vi "서보모터.vi"() -> ()   [LabVIEW 2018]
uses:
  <vilib>/DAQmx/write.llb/DAQmx Write (Counter Frequency 1Chan 1Samp).vi
  <vilib>/DAQmx/create/channels.llb/DAQmx Create Channel (CO-Pulse Generation-Frequency).vi
  <vilib>/DAQmx/configure/timing.llb/DAQmx Timing (Implicit).vi
  <vilib>/DAQmx/miscellaneous.llb/DAQmx Fill In Error Info.vi
panel:
  out "Duty Cycle":dbl
  in  "정지 버튼":bool
  in  "다이얼":dbl(knob)=0.5 caption="주기 점유율" scale=0.01..0.9
  in  "frequency":dbl=1.0 caption="주파수" format="%.6f"
  in  "initial delay":dbl caption="초기 지연" format="%.6f"
  in  "idle state":i32(ring)=10214 caption="유휴 상태" items=["하이"=10192, "로우"=10214]
  in  "counter":tag caption="카운터"
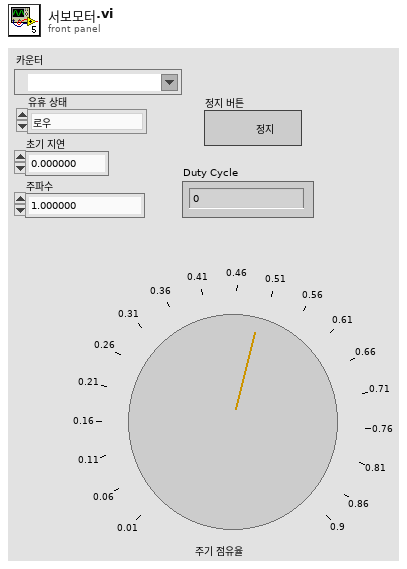
[diagram p1: front panel]
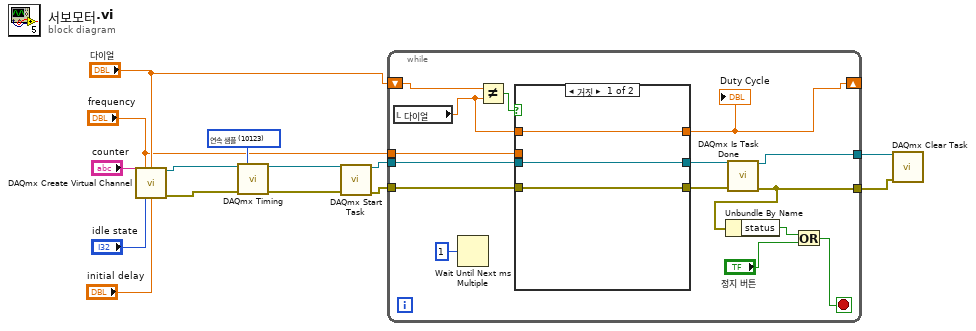
[diagram p0: block diagram]
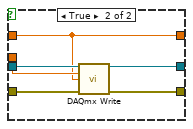
[diagram p2: hidden frame]
diagram:
  w7 = 10123 items=["유한 샘플"=10178, "연속 샘플"=10123, "하드웨어 타이밍에 의한 단일 포인트"=12522] ("sample mode")
  n1 = call-poly <vilib>:"DAQmx Create Virtual Channel.vi"("frequency"="frequency", "duty cycle"="다이얼", "counter"="counter", "idle state"="idle state", "initial delay"="initial delay") -> ("task out"=w14:refnum<k21>, "error out"=w13:errorcluster)  [unwired: 9 in]
  n2 = call-poly <vilib>:"DAQmx Timing.vi"("task/channels in"=w14, "sample mode"=w7, "error in"=w13) -> ("task out"=w11:refnum<k21>, "error out"=w12:errorcluster)  [unwired: 11 in]
  n3 = call <vilib>:"DAQmx Start Task.vi"("task/channels in"=w11, "error in"=w12) -> ("task out"=w4:refnum<k21>, "error out"=w3:errorcluster)  [unwired: 12 in]
  n4 = while {
    tunnel: [w29] -> w6
    tunnel: [w19] -> w5
    tunnel: w4 -> [w28]
    tunnel: w3 -> [w27]
    shift-right: [w21] -> _
    shift-left: "다이얼" -> [w24]
    tunnel: "frequency" -> [w20]
    stop <- w16 stop-if-true
    n5 = local read "다이얼"() -> (w22:dbl)
    n6 = Wait Until Next ms Multiple(millisecond multiple=u32 1 ("ms 배수")) -> ()  [unwired: 1 out]
    n7 = Not Equal?(x=w24, y=w22) -> (x != y?=w23:bool)
    n8 = case shown="거짓" w23 {
      tunnel: w28 -> [w32 w38]
      tunnel: w27 -> [w31 w37]
      tunnel: [w32 w36] -> w26
      tunnel: [w31 w35] -> w25
      tunnel: [w30 w33] -> w21
      tunnel: w22 -> [w30 w33]
      tunnel: w20 -> [_ w34]
      frame False {
      }
      frame True {
        n9 = call-poly <vilib>:"DAQmx Write.vi"("task/channels in"=w38, "frequency"=w34, "duty cycle"=w33, "error in"=w37) -> ("task out"=w36:refnum<k21>, "error out"=w35:errorcluster)  [unwired: 9 in, 1 out]
      }
    }
    "Duty Cycle" <- w21
    n10 = call <vilib>:"DAQmx Is Task Done.vi"("task/channels in"=w26, "error in"=w25) -> ("task out"=w29:refnum<k21>, "error out"=w19:errorcluster)  [unwired: 11 in, 1 out]
    n11 = Unbundle By Name(w19) -> ("status"=w18:bool)
    n12 = Or(x=w18, y="정지 버튼") -> (x .or. y?=w16:bool)
  }
  n13 = call <vilib>:"DAQmx Clear Task.vi"("task in"=w6, "error in"=w5) -> ()  [unwired: 13 in, 1 out]
